vi "host-C-Experimental-2.vi"() -> (0 "K(Indicator)":fxp<+/-,64,32>=1.52587890625e-05, 1 "degree":dbl=0.1952712924057206, 2 "Nominal Freq":fxp<+/-,64,32>=0.494873046875)   [LabVIEW 2012]
uses:
  <vilib>/FPGAPlugInAG/PCI-7831R/niLvFpga_Open_PCI-7831R.vi
  <vilib>/Utility/error.llb/Error Cluster From Error Code.vi
  <vilib>/rvi/errors/niLvFpgaAdjustHostInterfaceError.vi
  <vilib>/FPGAPlugInAG/PCI-7831R/niLvFpga_Abort_PCI-7831R.vi
  <vilib>/FPGAPlugInAG/PCI-7831R/niLvFpga_Close_PCI-7831R.vi
  <vilib>/FPGAPlugInAG/PCI-7831R/niLvFpga_Run_PCI-7831R.vi
  <vilib>/rvi/interface/common/dynamic/niFpgaDynamicAddResources.vi
  <vilib>/FPGAPlugInAG/Dynamic/niLvFpga_Close_Dynamic.vi
  <vilib>/Utility/file.llb/Write To Spreadsheet File (DBL).vi
  <vilib>/Utility/file.llb/Write To Spreadsheet File (I64).vi
  <vilib>/rvi/interface/nirviOpenFPGA/nirviOpenFPGA.xnode
  SB130-XPS/Documents/FPGA-project-apporach-retraction/FPGA Bitfiles/Apporach-Retract_FPGATarget_LIAFPGA-Experime_StHnuTKlnRU.lvbitx
  LIA_FPGA-Experimental-1.vi
  <vilib>/rvi/interface/nirviReadWriteControl/nirviReadWriteControl.xnode
  <vilib>/rvi/interface/nirviMethod/nirviMethod.xnode
  <vilib>/rvi/interface/nirviCloseFPGA/nirviCloseFPGA.xnode
  <vilib>/rvi/errors/niLvFpgaMergeErrorWithErrorCode.vi
  NiFpgaLv.dll
  <vilib>/FPGAPlugInAG/Dynamic/niLvFpga_StartFifo_Dynamic.vi
  <vilib>/FPGAPlugInAG/Dynamic/niLvFpga_StopFifo_Dynamic.vi
  <vilib>/FPGAPlugInAG/Dynamic/niLvFpga_ReadFifo_Dynamic.vi
panel:
  in  "Numeric 2":i32
  in  "Boolean":bool
  in  "Voltage":fxp<+/-,64,32>
  out "Corrected Frequency":fxp<+/-,64,32>
  out "Angular Frequency":fxp<+/-,64,32>
  out "Z":fxp<+/-,64,32>
  in  "Nominal Frequency":fxp<+/-,64,32>
  in  "VCO Constant":fxp<+/-,64,10>
  out "Waveform Chart 2":i32[](graph)
  out "Waveform Chart":i32[](graph)
  in  "Number of Elements":i32
  in  "Proportional Gain":fxp<+/-,64,32>
  in  "Integral Gain":fxp<+/-,64,32>
  out "P+I Error":fxp<+/-,64,32>
  out "PID Input Error":dbl
  out "Phase (Degree) Shift":fxp<+/-,64,32>
  out "Numeric":fxp<+/-,64,32>
  out "For Proportional":fxp<+/-,64,32>
  in  "DAQ Acquisition Rate":i32
  in  "Path 5":path
  in  "name-file 11":string="approach-15a"
  out "String 11":string
  in  "Path 7":path
  in  "name-file 9":string="approach-15a"
  out "String 9":string
  in  "Path 4":path
  in  "name-file 4":string="approach-15a"
  out "String 4":string
  in  "Path 3":path
  in  "name-file 3":string="approach-15a"
  out "String 3":string
  in  "Path 2":path
  in  "name-file 2":string="approach-15a"
  out "String 2":string
  in  "Data Collector":bool
  out "String":string
  in  "name-file":string="approach-15a"
  in  "Path":path
  out "Standardized nominal freq":dbl
  in  "Delta Nominal Frequency":dbl
  out "Ref":i32
  out "Sig":i32
  out "Sin":dbl(graph)
  out "Phase":dbl
  out "Ze Output":dbl=2.3841857910156248e-12
  out "The Decs":dbl=7.8125e-09
  out "LSB Weight":dbl=0.00030517578125
  in  "K":fxp<+,16,0>=1.52587890625e-05
  in  "nominal freq 2":fxp<+,16,0>=0.494873046875
  out "x*y":dbl=0.015
  in  "stop 2":bool
  out "3rd stages":i32=1
  out "3rd decimation":i32=977
  out "1st decimation":i32=1
  out "2nd decimation":i32=128
  in  "Time Constant [s]":dbl=2.5 min=0.0 step=0.0001 format="%.2f"
  in  "Filter Rolloff":enum16{"20 dB", "40 dB", "60 dB", "80 dB"}(ring)
  out "Actual Sampling Frequency":dbl=200000.0
  in  "input range of 9205":dbl=10.0
  in  "Sampling Frequency":dbl=200000.0 min=1000.0 max=250000.0
  in  "stop":bool
  out "r":dbl(graph)=0.5098420210496609
  out "y":dbl=0.0017376029872894286
  out "x":dbl=0.5098390600609779
  out "f":dbl(graph)=31000.332441180944
  in  "dec2":i16=1
  in  "nominal freq":dbl=30000.0 min=500.0 max=125000.0
  in  "dec1":i16=1000
  in  "stages":i8=1 min=1 max=2
  in  "decimation":i16=1000
  # "Sampling Frequency"
  # "CIC First Decimation"
  # "MA Stages"
  # "CIC Second Decimation"
  # "PLL Nominal Frequency"
  # "MA Decimation"
  # "PLL Frequency Output"
  # "LIA Output"
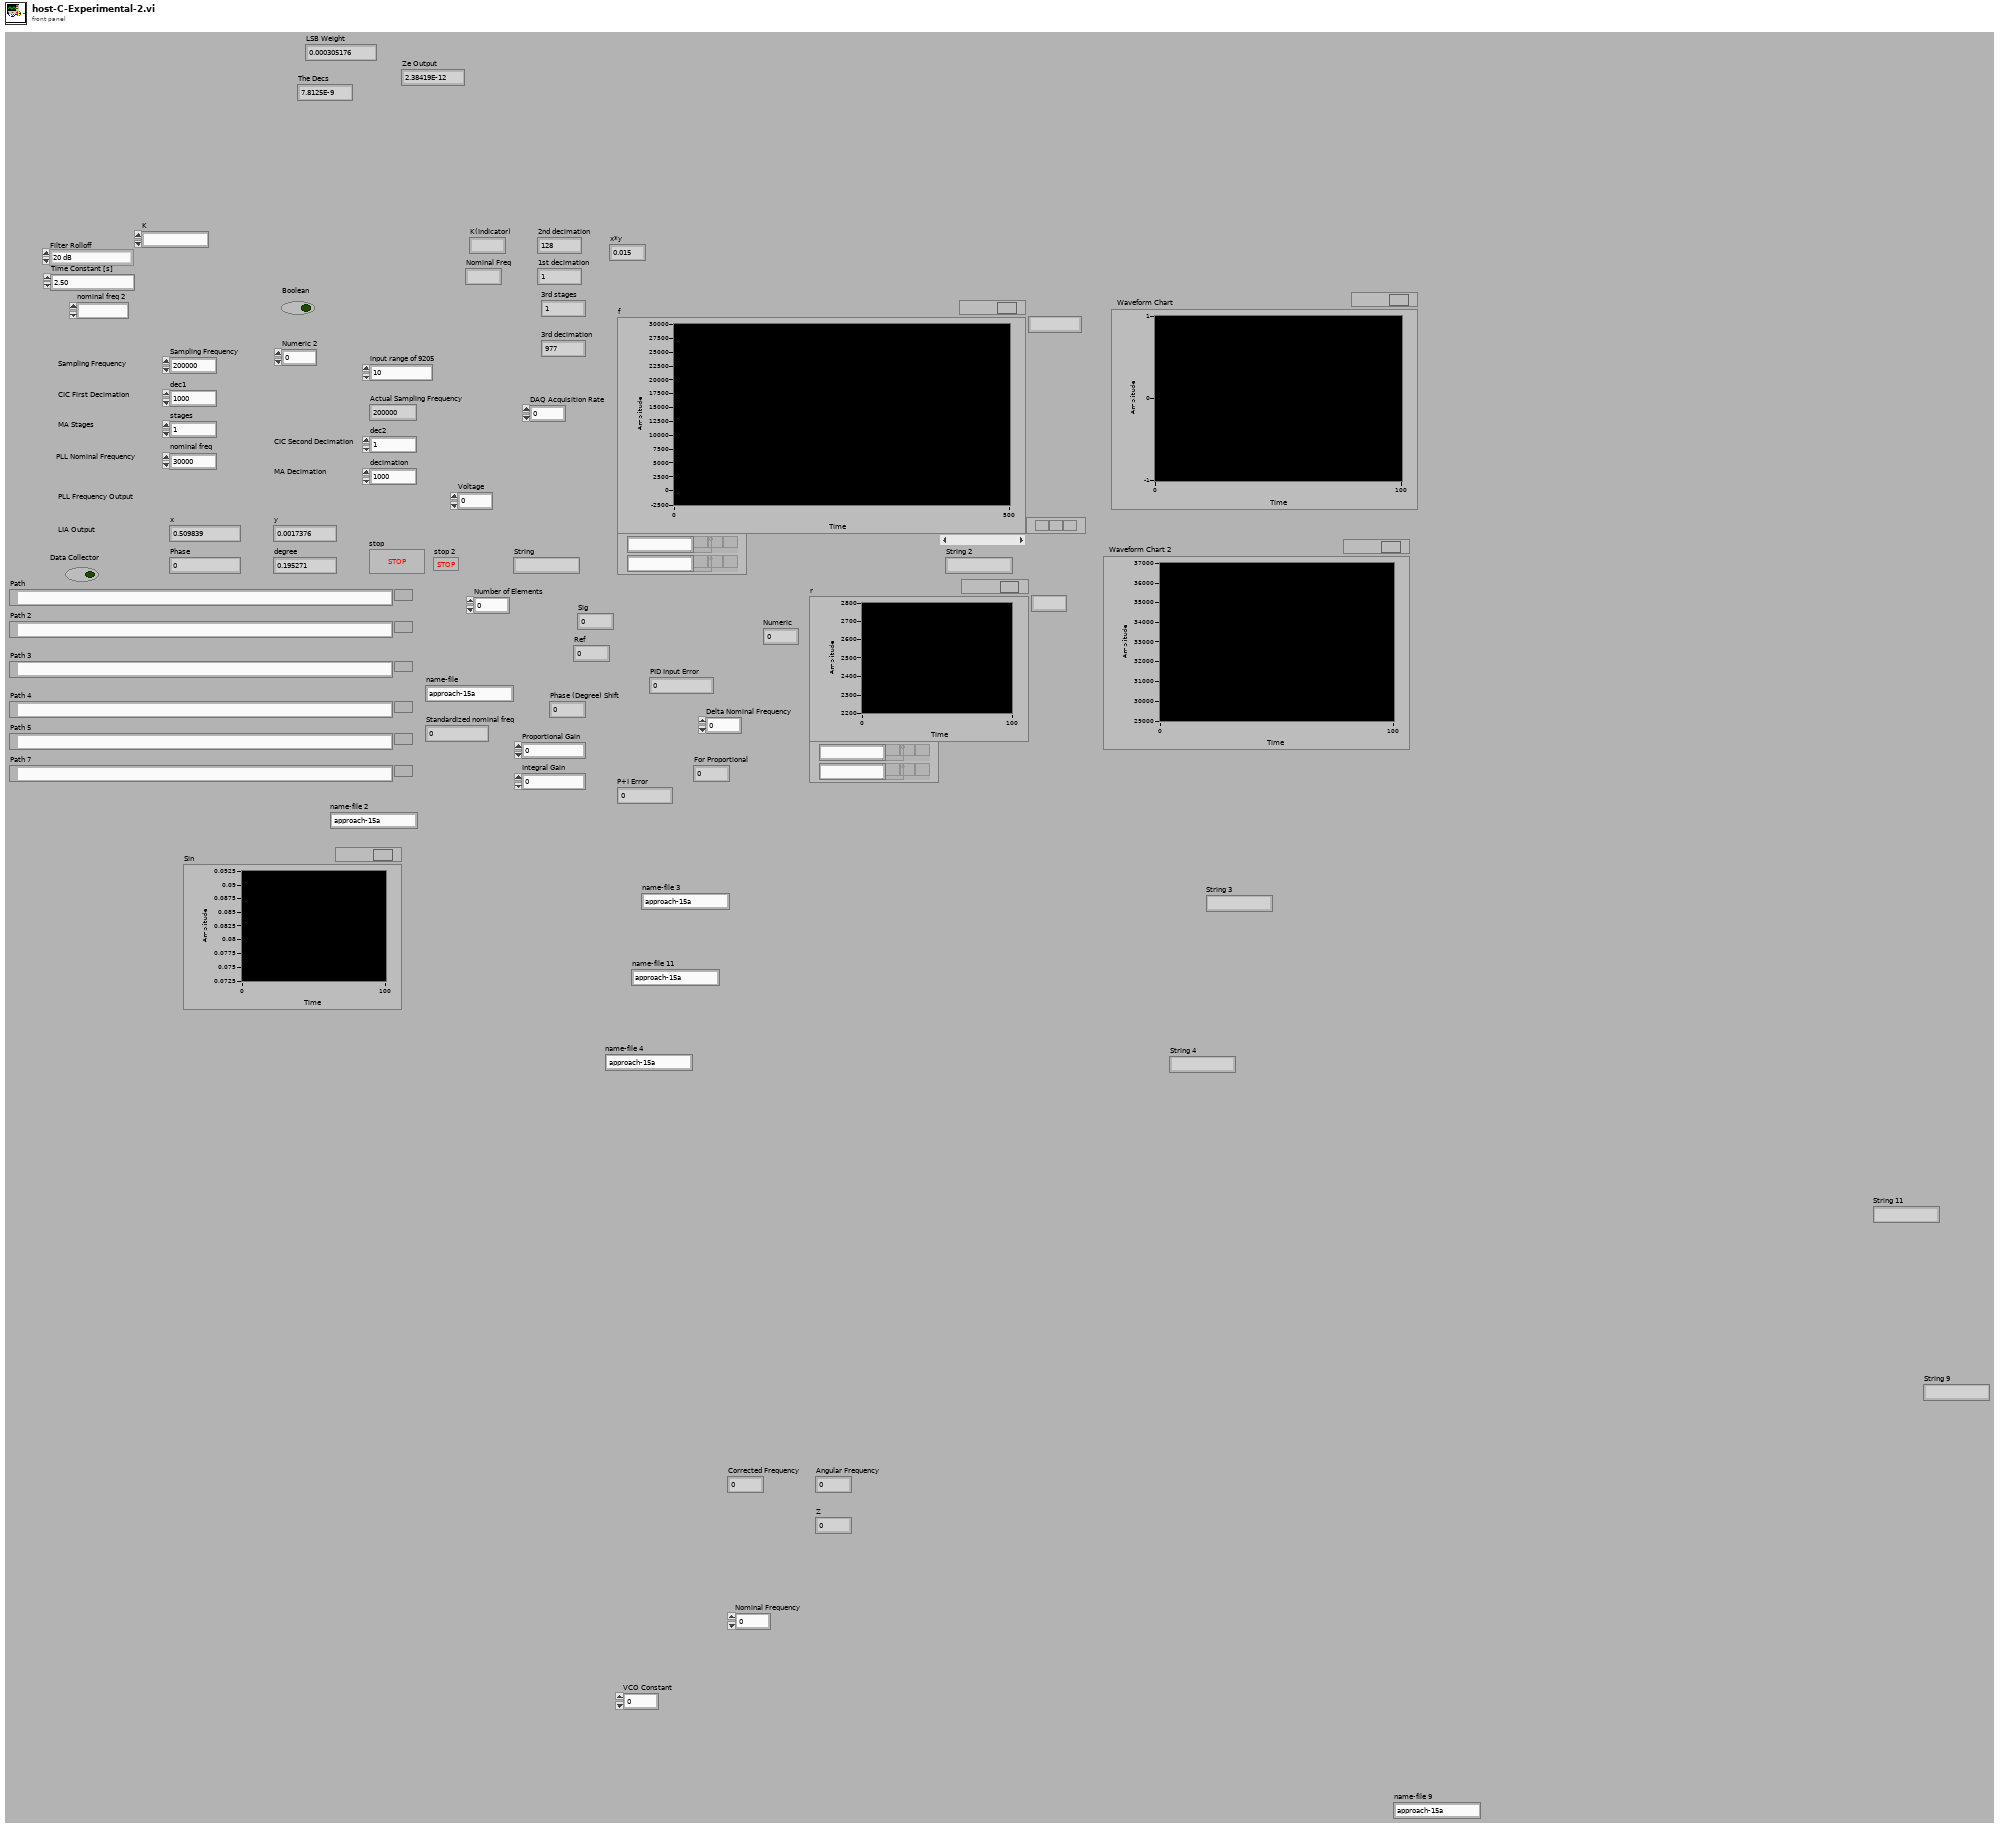
[diagram p1: front panel]
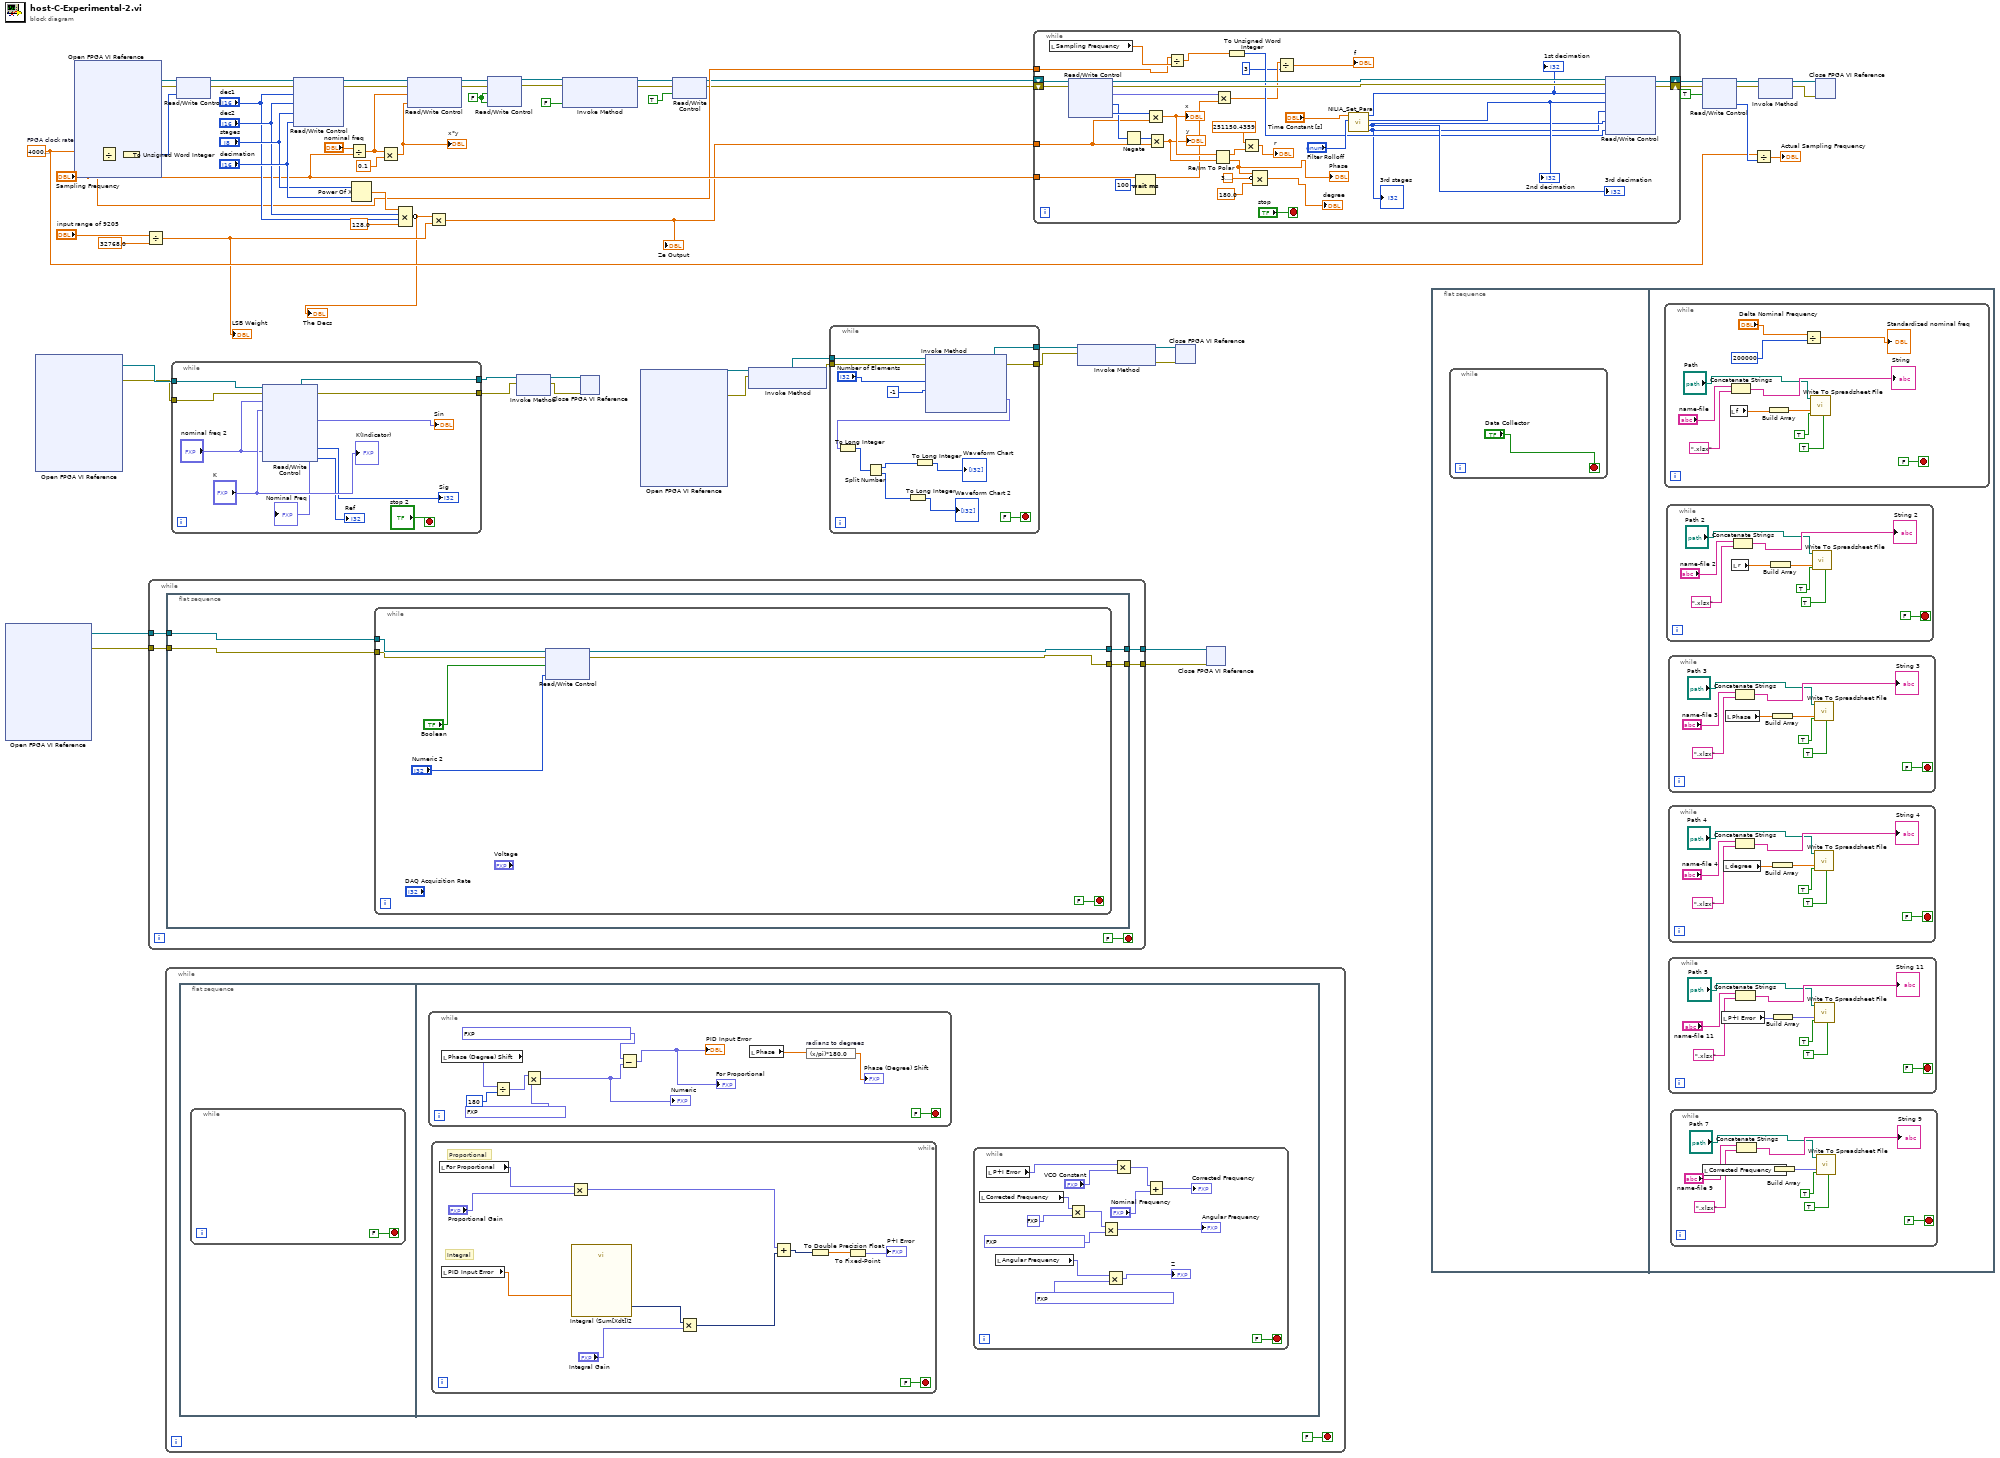
[diagram p0: block diagram]
diagram:
  w2 = FALSE
  w33 = 40000000.0  # FPGA clock rate
  n1 = xnode "Open FPGA VI Reference"() -> ("FPGA VI Reference Out"=w20:refnum<k20>, "error out"=w19:errorcluster)  [unwired: 2 in]
  n2 = xnode "Open FPGA VI Reference"() -> ("FPGA VI Reference Out"=w32:refnum<k20>, "error out"=w31:errorcluster)  [unwired: 2 in]
  n3 = xnode "Open FPGA VI Reference"() -> ("FPGA VI Reference Out"=w39:refnum<k20>, "error out"=w38:errorcluster)  [unwired: 2 in]
  n4 = Divide(x=w33, y="Sampling Frequency") -> (x/y=w45:dbl)
  n5 = To Unsigned Word Integer(number=w45) -> (unsigned 16bit integer=w44:u16)
  n6 = Divide(x="input range of 9205", y=32768.0) -> (x/y=w25:dbl)
  "LSB Weight" <- w25
  n7 = while {
    tunnel: [w67] -> w22
    tunnel: [w66] -> w21
    tunnel: w20 -> [w65]
    tunnel: w19 -> [w64]
    stop <- FALSE stop-if-true
    n8 = flat-sequence {
      tunnel: [w72] -> w67
      tunnel: [w71] -> w66
      tunnel: w64 -> [w69]
      tunnel: w65 -> [w70]
      frame #0 {
        n9 = while {
          tunnel: [w77] -> w72
          tunnel: [w76] -> w71
          tunnel: w70 -> [w79]
          tunnel: w69 -> [w78]
          stop <- FALSE stop-if-true
          n10 = xnode "Read/Write Control"("FPGA VI Reference In"=w79, "error in"=w78, "VCO Start"="Boolean", "Test"="Numeric 2") -> ("FPGA VI Reference Out"=w77:refnum<k20>, "error out"=w76:errorcluster)
        }
      }
    }
  }
  n11 = while {
    stop <- FALSE stop-if-true
    n12 = flat-sequence {
      frame #0 {
        n13 = while {
          stop <- FALSE stop-if-true
        }
      }
      frame #1 {
        n14 = while {
          stop <- FALSE stop-if-true
          n15 = local read "Phase (Degree) Shift"() -> (w96:fxp<+/-,64,32>)
          n16 = Divide(x=w96, y=i16 180) -> (x/y=w104:fxp<+/-,64,33>)
          n17 = Multiply(x=w104, y=fxp<+,30,2> 3.1415926814079285) -> (x*y=w103:fxp<+/-,64,35>)
          "Numeric" <- w103
          n18 = Subtract(x=fxp<+,50,1> 1.5707963199999995, y=w103) -> (x-y=→"PID Input Error" →"For Proportional":fxp<+/-,64,36>)
          n19 = local read "Phase"() -> (w98:dbl)
          n20 = expression code="(x/pi)*180.0" "radians to degrees"(w98) -> (→"Phase (Degree) Shift":dbl)
        }
        n21 = while {
          stop <- FALSE stop-if-true
          # "Integral"
          # "Proportional"
          n22 = local read "For Proportional"() -> (w116:fxp<+/-,64,32>)
          n23 = local read "PID Input Error"() -> (w114:dbl)
          n24 = Multiply(x=w116, y="Proportional Gain") -> (x*y=w111:fxp<+/-,64,64>)
          n25 = call "Integral (Sum[Xdt])2"("Signals"=w114) -> ("Result"=w113:dynamicdata)  [unwired: 5 in, 1 out]
          n26 = Multiply(x=w113, y="Integral Gain") -> (x*y=w110:dynamicdata)
          n27 = Add(x=w111, y=w110) -> (x+y=w109:dynamicdata)
          n28 = To Double Precision Float(number=w109) -> (double precision float=w108:dbl)
          n29 = To Fixed-Point(number=w108) -> (fixed-point=→"P+I Error":fxp<+/-,32,16>)  [unwired: 1 in]
        }
        n30 = while {
          stop <- FALSE stop-if-true
          n31 = local read "Corrected Frequency"() -> (w87:fxp<+/-,64,32>)
          n32 = local read "P+I Error"() -> (w82:fxp<+/-,64,32>)
          n33 = local read "Angular Frequency"() -> (w92:fxp<+/-,64,32>)
          n34 = Multiply(x=w87, y=fxp<+,1,2> 2.0) -> (x*y=w90:fxp<+/-,64,33>)
          n35 = Multiply(x=w90, y=fxp<+,30,2> 3.1415926814079285) -> (x*y=→"Angular Frequency":fxp<+/-,64,35>)
          n36 = Multiply(x=w92, y=fxp<+,46,7> 1.0000003385357559e-06) -> (x*y=→"Z":fxp<+/-,64,39>)
          n37 = Multiply(x=w82, y="VCO Constant") -> (x*y=w84:fxp<+/-,64,42>)
          n38 = Add(x=w84, y="Nominal Frequency") -> (x+y=→"Corrected Frequency":fxp<+/-,64,43>)
        }
      }
    }
  }
  n39 = while {
    tunnel: w32 -> [w125]
    tunnel: w31 -> [w124]
    tunnel: [w123] -> w30
    tunnel: [w122] -> w29
    stop <- "stop 2" stop-if-true
    n40 = xnode "Read/Write Control"("FPGA VI Reference In"=w125, "error in"=w124, "nominal freq"="nominal freq 2", "K"="K") -> ("FPGA VI Reference Out"=w123:refnum<k20>, "error out"=w122:errorcluster, "Sin"=→"Sin":fxp<+/-,14,2>, "sig"=→"Sig":i16, "ref"=→"Ref":i16)  [unwired: 2 out]
    "K(Indicator)" <- "K"
    "Nominal Freq" <- "nominal freq 2"
  }
  n41 = xnode "Read/Write Control"("FPGA VI Reference In"=w39, "error in"=w38, "Period"=w44) -> ("FPGA VI Reference Out"=w47:refnum<k20>, "error out"=w46:errorcluster)
  n42 = xnode "Read/Write Control"("FPGA VI Reference In"=w47, "error in"=w46, "dec1"="dec1", "dec2"="dec2", "stages"="stages", "decimation"="decimation") -> ("FPGA VI Reference Out"=w63:refnum<k20>, "error out"=w62:errorcluster)
  n43 = Divide(x="nominal freq", y="Sampling Frequency") -> (x/y=w41:dbl)
  n44 = Power Of X(1:"decimation", 2:"stages") -> (0:w58:dbl)
  n45 = Multiply(x=w41, y=0.1) -> (x*y=w26:dbl)
  "x*y" <- w26
  n46 = Compound Arithmetic op=MULTIPLY(w58, "dec2", "dec1", 128.0) -> (invert w24:dbl)
  "The Decs" <- w24
  n47 = xnode "Read/Write Control"("FPGA VI Reference In"=w63, "error in"=w62, "nominal freq"=w41, "K"=w26) -> ("FPGA VI Reference Out"=w6:refnum<k20>, "error out"=w4:errorcluster)
  n48 = Multiply(x=w24, y=w25) -> (x*y=w23:dbl)
  "Ze Output" <- w23
  n49 = xnode "Read/Write Control"("FPGA VI Reference In"=w6, "error in"=w4, "start"=w2, "stop"=w2) -> ("FPGA VI Reference Out"=w5:refnum<k20>, "error out"=w3:errorcluster)
  n50 = xnode "Invoke Method"("FPGA VI Reference In"=w30, "error in"=w29) -> ("FPGA VI Reference Out"=w28:refnum<k20>, "error out"=w27:errorcluster)
  n51 = xnode "Invoke Method"("FPGA VI Reference In"=w5, "error in"=w3, "Wait Until Done (F)"=FALSE) -> ("FPGA VI Reference Out"=w10:refnum<k20>, "error out"=w9:errorcluster)
  n52 = xnode "Close FPGA VI Reference"("FPGA VI Reference In"=w28, "error in"=w27) -> ()  [unwired: 1 out]
  n53 = xnode "Open FPGA VI Reference"() -> ("FPGA VI Reference Out"=w18:refnum<k20>, "error out"=w17:errorcluster)  [unwired: 2 in]
  n54 = xnode "Read/Write Control"("FPGA VI Reference In"=w10, "error in"=w9, "start"=TRUE) -> ("FPGA VI Reference Out"=w8:refnum<k20>, "error out"=w7:errorcluster)
  n55 = xnode "Invoke Method"("FPGA VI Reference In"=w18, "error in"=w17) -> ("FPGA VI Reference Out"=w16:refnum<k20>, "error out"=w15:errorcluster)
  n56 = while {
    tunnel: w16 -> [w134]
    tunnel: w15 -> [w133]
    tunnel: [w132] -> w12
    tunnel: [w131] -> w11
    stop <- FALSE stop-if-true
    n57 = xnode "Invoke Method"("FPGA VI Reference In"=w134, "error in"=w133, "Number of Elements"="Number of Elements", "Timeout (ms)"=-1) -> ("FPGA VI Reference Out"=w132:refnum<k20>, "error out"=w131:errorcluster, "Data"=w127:fxp<+/-,64,16>[])  [unwired: 1 out]
    n58 = To Long Integer(number=w127) -> (32bit integer=w130:i32[])
    n59 = Split Number(x=w130) -> (hi(x)=w138:u16[], lo(x)=w137:u16[])
    n60 = To Long Integer(number=w137) -> (32bit integer=→"Waveform Chart 2":i32[])
    n61 = To Long Integer(number=w138) -> (32bit integer=→"Waveform Chart":i32[])
  }
  n62 = while {
    shift-right: [w159] -> w54
    shift-left: w8 -> [w173]
    shift-right: [w158] -> w53
    shift-left: w7 -> [w172]
    tunnel: w23 -> [w169]
    tunnel: "Sampling Frequency" -> [w161]
    tunnel: w33 -> [w151]
    stop <- "stop" stop-if-true
    n63 = local read "Sampling Frequency"() -> (w152:dbl)
    n64 = xnode "Read/Write Control"("FPGA VI Reference In"=w173, "error in"=w172) -> ("FPGA VI Reference Out"=w159:refnum<k20>, "error out"=w158:errorcluster, "f"=w162:fxp<+/-,32,0>, "channelQ"=w170:i64, "channelI"=w171:i64)
    n65 = Negate(x=w170) -> (-x=w160:i64)
    n66 = Wait (ms)(milliseconds to wait=u32 100) -> ()  [unwired: 1 out]
    n67 = Multiply(x=w171, y=w169) -> (x*y=w168:dbl)
    "x" <- w168
    n68 = Multiply(x=w160, y=w169) -> (x*y=w167:dbl)
    "y" <- w167
    n69 = Divide(x=w151, y=w152) -> (x/y=w150:dbl)
    n70 = Re/Im To Polar(2:w167, 3:w168) -> (0:w143:dbl, 1:w146:dbl)
    "Phase" <- w143
    n71 = Multiply(x=w162, y=w161) -> (x*y=w142:dbl)
    n72 = To Unsigned Word Integer(number=w150) -> (unsigned 16bit integer=w149:u16)
    n73 = Multiply(x=251150.4359, y=w146) -> (x*y=→"r":dbl)
    n74 = Compound Arithmetic op=MULTIPLY(w143, invert 3.141592653589793, 180.0 ("value")) -> (→"degree":dbl)
    n75 = Divide(x=w142, y=3) -> (x/y=→"f":dbl)
    n76 = call "NILIA_Set_Para.vi"("rolloff"="Filter Rolloff", "TC [sec]"="Time Constant [s]") -> ("3rd stages"=w148:i32, "3rd decimation"=w153:i32, "2nd decimation"=w154:i32, "1st decimation"=w155:i32)  [unwired: 5 in, 1 out]
    "2nd decimation" <- w154
    "1st decimation" <- w155
    "3rd decimation" <- w153
    "3rd stages" <- w148
    n77 = xnode "Read/Write Control"("FPGA VI Reference In"=w159, "error in"=w158, "dec1"=w155, "dec2"=w154, "stages"=w148, "decimation"=w153, "Period"=w149) -> ()  [unwired: 2 out]
  }
  n78 = xnode "Invoke Method"("FPGA VI Reference In"=w12, "error in"=w11) -> ("FPGA VI Reference Out"=w14:refnum<k20>, "error out"=w13:errorcluster)
  n79 = xnode "Close FPGA VI Reference"("FPGA VI Reference In"=w14, "error in"=w13) -> ()  [unwired: 1 out]
  n80 = xnode "Close FPGA VI Reference"("FPGA VI Reference In"=w22, "error in"=w21) -> ()  [unwired: 1 out]
  n81 = flat-sequence {
    frame #0 {
      n82 = while {
        stop <- "Data Collector" stop-if-true
      }
    }
    frame #1 {
      n83 = while {
        stop <- FALSE stop-if-true
        n84 = local read "f"() -> (w227:dbl)
        n85 = Concatenate Strings("name-file", ".xlsx") -> (→"String":string)
        n86 = Build Array(w227) -> (w226:dbl[])
        n87 = Divide(x="Delta Nominal Frequency", y=200000) -> (x/y=→"Standardized nominal freq":dbl)
        n88 = call-poly <vilib>:"Write To Spreadsheet File.vi"("transpose? (no:F)"=TRUE, "append to file? (new file:F)"=TRUE, "1D data"=w226, "file path (dialog if empty)"="Path") -> ()  [unwired: 4 in, 1 out]
      }
      n89 = while {
        stop <- FALSE stop-if-true
        n90 = local read "r"() -> (w218:dbl)
        n91 = Concatenate Strings("name-file 2", ".xlsx") -> (→"String 2":string)
        n92 = Build Array(w218) -> (w217:dbl[])
        n93 = call-poly <vilib>:"Write To Spreadsheet File.vi"("transpose? (no:F)"=TRUE, "append to file? (new file:F)"=TRUE, "1D data"=w217, "file path (dialog if empty)"="Path 2") -> ()  [unwired: 4 in, 1 out]
      }
      n94 = while {
        stop <- FALSE stop-if-true
        n95 = local read "Phase"() -> (w209:dbl)
        n96 = Concatenate Strings("name-file 3", ".xlsx") -> (→"String 3":string)
        n97 = Build Array(w209) -> (w208:dbl[])
        n98 = call-poly <vilib>:"Write To Spreadsheet File.vi"("transpose? (no:F)"=TRUE, "append to file? (new file:F)"=TRUE, "1D data"=w208, "file path (dialog if empty)"="Path 3") -> ()  [unwired: 4 in, 1 out]
      }
      n99 = while {
        stop <- FALSE stop-if-true
        n100 = local read "degree"() -> (w200:dbl)
        n101 = Concatenate Strings("name-file 4", ".xlsx") -> (→"String 4":string)
        n102 = Build Array(w200) -> (w199:dbl[])
        n103 = call-poly <vilib>:"Write To Spreadsheet File.vi"("transpose? (no:F)"=TRUE, "append to file? (new file:F)"=TRUE, "1D data"=w199, "file path (dialog if empty)"="Path 4") -> ()  [unwired: 4 in, 1 out]
      }
      n104 = while {
        stop <- FALSE stop-if-true
        n105 = local read "P+I Error"() -> (w182:fxp<+/-,64,32>)
        n106 = Concatenate Strings("name-file 11", ".xlsx") -> (→"String 11":string)
        n107 = Build Array(w182) -> (w181:fxp<+/-,64,32>[])
        n108 = call-poly <vilib>:"Write To Spreadsheet File.vi"("transpose? (no:F)"=TRUE, "append to file? (new file:F)"=TRUE, "1D data"=w181, "file path (dialog if empty)"="Path 5") -> ()  [unwired: 4 in, 1 out]
      }
      n109 = while {
        stop <- FALSE stop-if-true
        n110 = local read "Corrected Frequency"() -> (w191:fxp<+/-,64,32>)
        n111 = Concatenate Strings("name-file 9", ".xlsx") -> (→"String 9":string)
        n112 = Build Array(w191) -> (w190:fxp<+/-,64,32>[])
        n113 = call-poly <vilib>:"Write To Spreadsheet File.vi"("transpose? (no:F)"=TRUE, "append to file? (new file:F)"=TRUE, "1D data"=w190, "file path (dialog if empty)"="Path 7") -> ()  [unwired: 4 in, 1 out]
      }
    }
  }
  n114 = xnode "Read/Write Control"("FPGA VI Reference In"=w54, "error in"=w53, "stop"=TRUE) -> ("FPGA VI Reference Out"=w51:refnum<k20>, "error out"=w50:errorcluster, "ticks"=w35:u32)
  n115 = Divide(x=w33, y=w35) -> (x/y=→"Actual Sampling Frequency":dbl)
  n116 = xnode "Invoke Method"("FPGA VI Reference In"=w51, "error in"=w50) -> ("FPGA VI Reference Out"=w49:refnum<k20>, "error out"=w48:errorcluster)
  n117 = xnode "Close FPGA VI Reference"("FPGA VI Reference In"=w49, "error in"=w48) -> ()  [unwired: 1 out]
